vi "Lift.vi"() -> ()   [LabVIEW 2018]
uses:
  <vilib>/Rock Robotics/SystemInterfaces/DIO/FPGA_DIOChannel.ctl
  <vilib>/Rock Robotics/WPI/ThirdParty/Phoenix-LabVIEW/Motor Controller/Controls/CTRE_Phoenix_MotorControl_ControlMode.ctl
  <vilib>/Rock Robotics/WPI/Counter/WPI_CounterDigitalInputToDigitalSource.vi
  Lift Global.vi
  Times/Times Global.vi
  Cargo Intake/Cargo Intake Global.vi
  <vilib>/addons/control/pid/pid.llb/PID (DBL).vi
  <vilib>/addons/control/pid/NI_PID_pid.lvlib
panel:
  in  "LiftMode":T1(ring)
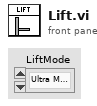
[diagram p1: front panel]
types:
  T1 = enum16{"Ultra Manual Control", "Manual Control", "Basic Control", "Automated Control", "Autonomous Control"}
  T2 = typedef "FPGA_DIOChannel.ctl" = enum8{"DIO 0", "DIO 1", "DIO 2", "DIO 3", "DIO 4", "DIO 5", "DIO 6", "DIO 7", "DIO 8", "DIO 9", "DIO MXP 0", "DIO MXP 1", "DIO MXP 2", "DIO MXP 3", "DIO MXP 4", "DIO MXP 5", "DIO MXP 6", "DIO MXP 7", "DIO MXP 8", "DIO MXP 9", "DIO MXP 10", "DIO MXP 11", "DIO MXP 12", "DIO MXP 13", "DIO MXP 14", "DIO MXP 15", "SPI Port CS1", "SPI Port CS2", "SPI Port CS3", "SPI Port MISO", "SPI Port MOSI", "Invalid"}
  T3 = typedef "WPI_DigitalInputDevRef.ctl" = cluster{"DevStatus":errorcluster, "DIO Channel":T2}
  T4 = enum16{"N/A", "Hatch Panel Zone 1", "Hatch Panel Zone 2", "Hatch Panel Zone 3", "Cargo Zone 1", "Cargo Zone 2", "Cargo Zone 3"}
  T5 = typedef "WPI_MotorControlDeviceRef.ctl" = cluster{"DeviceStatus":errorcluster, "Type":T6, "PWM":cluster{"PWM Channel":T7, "DeadBand":T8}, "CAN":cluster{"Device Number":u8, "SetOutput VI Ref":variant, "GetOutput VI Ref":variant, "Enable VI Ref":variant, "Disable VI Ref":variant, "Data":variant}, "Invert":bool, "DIO PWM":cluster{"PWM \"Enable\" Channel":T7, "DIOChannel":T2, "PWM Rate":dbl}}
  T6 = typedef "WPI_MotorControlType.ctl" = enum16{"PWM", "CAN", "DIO PWM"}
  T7 = typedef "FPGA_DIOPWMChannel.ctl" = enum8{"PWM 0", "PWM 1", "PWM 2", "PWM 3", "PWM 4", "PWM 5", "PWM 6", "PWM 7", "PWM 8", "PWM 9", "PWM MXP 0", "PWM MXP 1", "PWM MXP 2", "PWM MXP 3", "PWM MXP 4", "PWM MXP 5", "PWM MXP 6", "PWM MXP 7", "PWM MXP 8", "PWM MXP 9", "Invalid"}
  T8 = typedef "WPI_PWMDeadband.ctl" = cluster{"Name":string, "maxPositivePwm":i32, "minPositivePwm":i32, "centerPwm":i32, "maxNegativePwm":i32, "minNegativePwm":i32, "angularRange":u16}
  T9 = typedef "CTRE_Phoenix_MotorControl_ControlMode.ctl" = u16
  T10 = typedef "Control 3.ctl" = dbl
  T11 = cluster{"proportional gain (Kc)":dbl, "integral time(Ti, min)":dbl, "derivative time(Td, min) 2":dbl}
  T12 = typedef "FPGA_CounterEncoderSourceConvertionLVSourceType.ctl" = cluster{"DevStatus":errorcluster, "AnalogTriggerMode?":bool, "DigitalMode":cluster{"DIO Channel":T13}, "AnalogTriggerMode":cluster{"AnalogTriggerIndex":T14, "OutputType":T15}}
  T13 = typedef "FPGA_DIODigitalSourceChannel.ctl" = enum8{"DIO 0", "DIO 1", "DIO 2", "DIO 3", "DIO 4", "DIO 5", "DIO 6", "DIO 7", "DIO 8", "DIO 9", "DIO MXP 0", "DIO MXP 1", "DIO MXP 2", "DIO MXP 3", "DIO MXP 4", "DIO MXP 5", "DIO MXP 6", "DIO MXP 7", "DIO MXP 8", "DIO MXP 9", "DIO MXP 10", "DIO MXP 11", "DIO MXP 12", "DIO MXP 13", "DIO MXP 14", "DIO MXP 15", "SPI Port CS1", "SPI Port CS2", "SPI Port CS3", "SPI Port MISO", "SPI Port MOSI", "Disabled"}
  T14 = typedef "FPGA_AnalogTriggerIndex.ctl" = enum8{"Trig 0", "Trig 1", "Trig 2", "Trig 3", "Trig 4", "Trig 5", "Trig 6", "Trig 7", "Invalid"}
  T15 = typedef "FPGA_AnalogTriggerOutType.ctl" = enum16{"InWindow", "TriggerState", "Rising", "Falling"}
  T16 = typedef "WPI_EncoderDevRef.ctl" = cluster{"DevStatus":errorcluster, "EncoderIndex":T17, "CounterIndex":T18, "DistancePerCount":dbl, "Decoding Type":T19}
  T17 = typedef "FPGA_EncoderIdx.ctl" = enum8{"Enc 0", "Enc 1", "Enc 2", "Enc 3", "Enc 4", "Enc 5", "Enc 6", "Enc 7", "Invalid"}
  T18 = typedef "FPGA_CounterCtrSystemIndex.ctl" = enum8{"Ctr 0", "Ctr 1", "Ctr 2", "Ctr 3", "Ctr 4", "Ctr 5", "Ctr 6", "Ctr 7", "Invalid"}
  T19 = typedef "WPI_EncoderType.ctl" = enum16{"1x", "2x", "4x"}
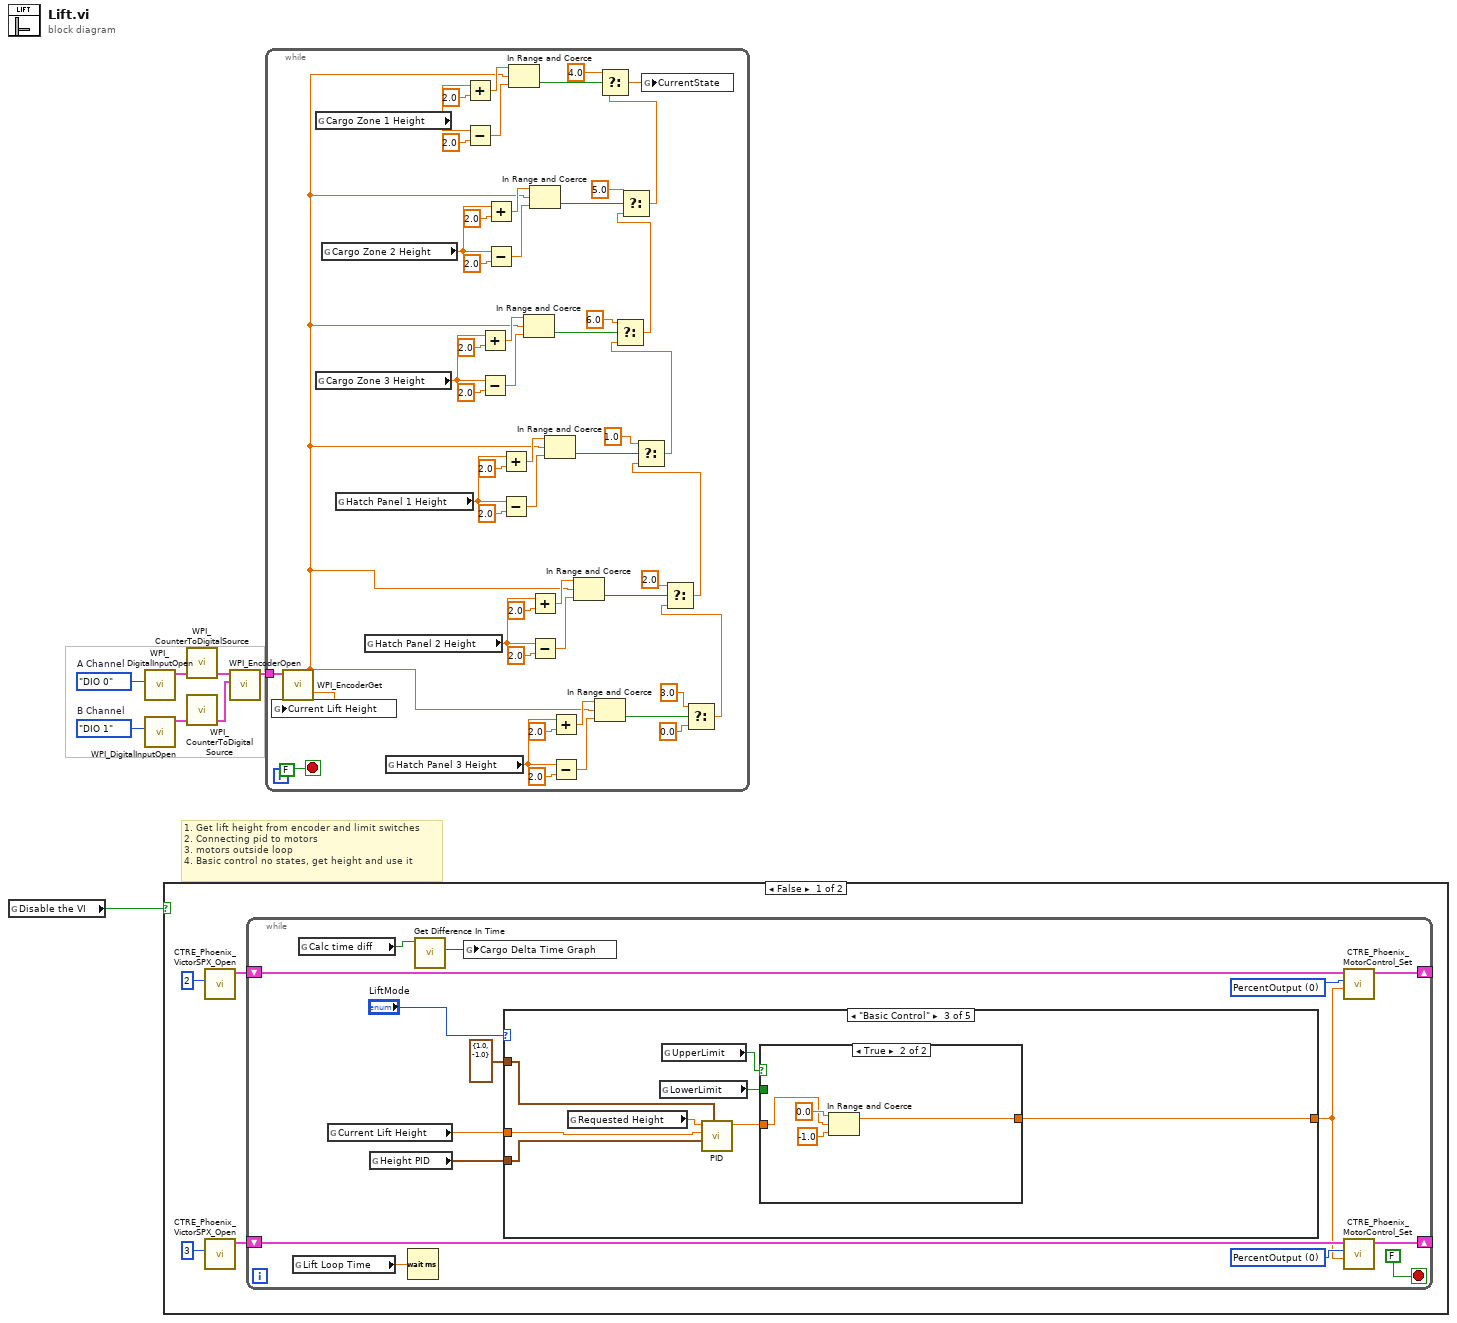
[diagram p0: block diagram]
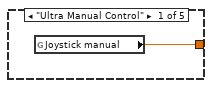
[diagram p2: hidden frame]
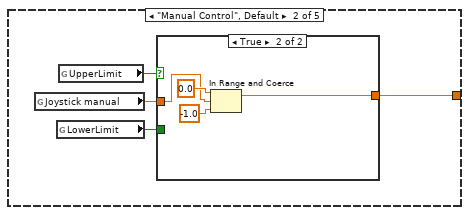
[diagram p3: hidden frame]
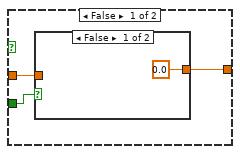
[diagram p4: hidden frame]
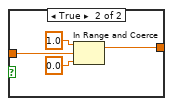
[diagram p5: hidden frame]
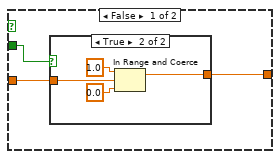
[diagram p6: hidden frame]
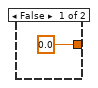
[diagram p7: hidden frame]
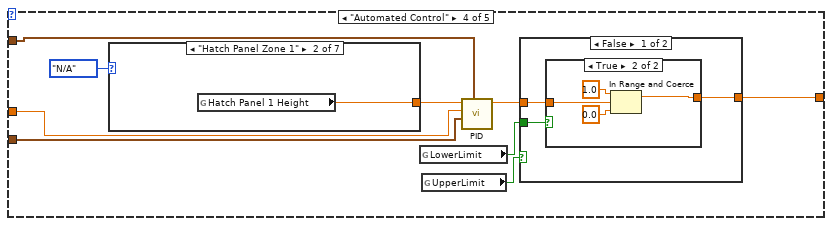
[diagram p8: hidden frame]
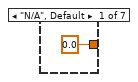
[diagram p9: hidden frame]
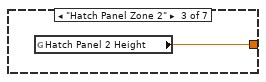
[diagram p10: hidden frame]
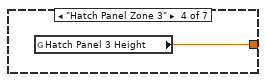
[diagram p11: hidden frame]
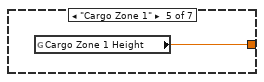
[diagram p12: hidden frame]
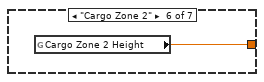
[diagram p13: hidden frame]
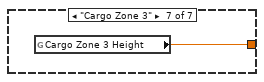
[diagram p14: hidden frame]
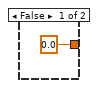
[diagram p15: hidden frame]
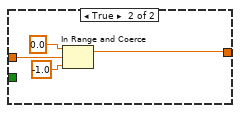
[diagram p16: hidden frame]
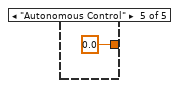
[diagram p17: hidden frame]
diagram:
  w8 = FPGA_DIOChannel."DIO 1"  # B Channel
  w7 = FPGA_DIOChannel."DIO 0"  # A Channel
  # "1. Get lift height from encoder and limit switches\n2. Connecting pid to motors\n3. motors outside loop\n4. Basic control no states, get height and use it"
  n1 = global read "Lift Global.vi" "Disable the VI"() -> (w1:bool)
  n2 = call <vilib>:"WPI_DigitalInputOpen.vi"("DIO Channel"=w7) -> ("DigitalInputDevRef"=w4:T3)  [unwired: 1 in, 9 out]
  n3 = call <vilib>:"WPI_DigitalInputOpen.vi"("DIO Channel"=w8) -> ("DigitalInputDevRef"=w5:T3)  [unwired: 1 in, 9 out]
  n4 = case shown="False" w1 {
    frame False {
      n5 = call <vilib>:"CTRE_Phoenix_VictorSPX_Open.vi"("Device Number"=u8 2) -> ("CAN Talon SRX Ref"=w12:T5)  [unwired: 9 in, 1 out]
      n6 = call <vilib>:"CTRE_Phoenix_VictorSPX_Open.vi"("Device Number"=u8 3) -> ("CAN Talon SRX Ref"=w10:T5)  [unwired: 9 in, 1 out]
      n7 = while {
        shift-right: [w21] -> _
        shift-left: w12 -> [w18]
        shift-right: [w19] -> _
        shift-left: w10 -> [w17]
        stop <- FALSE stop-if-true
        w20 = T9 0 items=["PercentOutput"=0, "Position"=1, "Velocity"=2, "Current"=3, "Follower"=5, "MotionProfile"=6, "MotionMagic"=7, "MotionProfileArc"=10, "Disabled"=15] ("Control Mode")
        w22 = T9 0 items=["PercentOutput"=0, "Position"=1, "Velocity"=2, "Current"=3, "Follower"=5, "MotionProfile"=6, "MotionMagic"=7, "MotionProfileArc"=10, "Disabled"=15] ("Control Mode")
        n8 = global read "Times Global.vi" "Lift Loop Time"() -> (w27:T10)
        n9 = global read "Cargo Intake Global.vi" "Calc time diff"() -> (w24:bool)
        n10 = global read "Lift Global.vi" "Current Lift Height"() -> (w13:dbl)
        n11 = global read "Lift Global.vi" "Height PID"() -> (w14:T11)
        n12 = Wait (ms)(milliseconds to wait=w27) -> ()  [unwired: 1 out]
        n13 = call "Get Difference In Time.vi"("Calculate Time Difference"=w24) -> ("Delta Time over Time"=w23:u32)  [unwired: 9 in, 1 out]
        n14 = global write "Times Global.vi" "Cargo Delta Time Graph"(w23) -> ()
        n15 = case shown="\"Basic Control\"" "LiftMode" {
          tunnel: [w28 w29 w46 w70 0.0 ("Cargo Zone 3 Height")] -> w16
          tunnel: w13 -> [_ _ w52 w68 _]
          tunnel: w14 -> [_ _ w51 w67 _]
          tunnel: cluster{"output high":dbl, "output low":dbl} {"output high"=1.0, "output low"=-1.0} ("output range") -> [_ _ w50 w69 _]
          frame "Ultra Manual Control" {
            n16 = global read "Lift Global.vi" "Joystick manual"() -> (w28:dbl)
          }
          frame "Manual Control", Default {
            n17 = global read "Lift Global.vi" "Joystick manual"() -> (w30:dbl)
            n18 = global read "Lift Global.vi" "LowerLimit"() -> (w32:bool)
            n19 = global read "Lift Global.vi" "UpperLimit"() -> (w31:bool)
            n20 = case shown="True" w31 {
              tunnel: w32 -> [w35 _]
              tunnel: [w34 w42] -> w29
              tunnel: w30 -> [w33 w41]
              frame False {
                n21 = case shown="False" w35 {
                  tunnel: [0.0 w40] -> w34
                  tunnel: w33 -> [_ w37]
                  frame False {
                  }
                  frame True {
                    n22 = In Range and Coerce(upper limit=1.0, x=w37, lower limit=0.0) -> (coerced(x)=w40:dbl)  [unwired: 1 out]
                  }
                }
              }
              frame True {
                n23 = In Range and Coerce(upper limit=0.0, x=w41, lower limit=-1.0) -> (coerced(x)=w42:dbl)  [unwired: 1 out]
              }
            }
          }
          frame "Basic Control" {
            n24 = global read "Lift Global.vi" "Requested Height"() -> (w45:dbl)
            n25 = global read "Lift Global.vi" "LowerLimit"() -> (w49:bool)
            n26 = global read "Lift Global.vi" "UpperLimit"() -> (w48:bool)
            n27 = call-poly <vilib>:"PID.vi"("output range"=w50, "PID gains"=w51, "process variable"=w52, "setpoint"=w45) -> ("output"=w47:dbl)  [unwired: 6 in, 1 out]
            n28 = case shown="True" w48 {
              tunnel: w49 -> [w55 _]
              tunnel: [w54 w62] -> w46
              tunnel: w47 -> [w53 w61]
              frame False {
                n29 = case shown="True" w55 {
                  tunnel: [0.0 w60] -> w54
                  tunnel: w53 -> [_ w57]
                  frame False {
                  }
                  frame True {
                    n30 = In Range and Coerce(upper limit=1.0, x=w57, lower limit=0.0) -> (coerced(x)=w60:dbl)  [unwired: 1 out]
                  }
                }
              }
              frame True {
                n31 = In Range and Coerce(upper limit=0.0, x=w61, lower limit=-1.0) -> (coerced(x)=w62:dbl)  [unwired: 1 out]
              }
            }
          }
          frame "Automated Control" {
            n32 = case shown="\"Hatch Panel Zone 1\"" T4."N/A" ("LiftLocation") {
              tunnel: [0.0 ("Cargo Zone 3 Height") w75 w76 w77 w78 w79 w80] -> w65
              frame "N/A", Default {
              }
              frame "Hatch Panel Zone 1" {
                n33 = global read "Lift Global.vi" "Hatch Panel 1 Height"() -> (w75:dbl)
              }
              frame "Hatch Panel Zone 2" {
                n34 = global read "Lift Global.vi" "Hatch Panel 2 Height"() -> (w76:dbl)
              }
              frame "Hatch Panel Zone 3" {
                n35 = global read "Lift Global.vi" "Hatch Panel 3 Height"() -> (w77:dbl)
              }
              frame "Cargo Zone 1" {
                n36 = global read "Lift Global.vi" "Cargo Zone 1 Height"() -> (w78:dbl)
              }
              frame "Cargo Zone 2" {
                n37 = global read "Lift Global.vi" "Cargo Zone 2 Height"() -> (w79:dbl)
              }
              frame "Cargo Zone 3" {
                n38 = global read "Lift Global.vi" "Cargo Zone 3 Height"() -> (w80:dbl)
              }
            }
            n39 = global read "Lift Global.vi" "LowerLimit"() -> (w73:bool)
            n40 = global read "Lift Global.vi" "UpperLimit"() -> (w72:bool)
            n41 = call-poly <vilib>:"PID.vi"("output range"=w69, "PID gains"=w67, "process variable"=w68, "setpoint"=w65) -> ("output"=w71:dbl)  [unwired: 6 in, 1 out]
            n42 = case shown="False" w72 {
              tunnel: w73 -> [w83 _]
              tunnel: [w82 w90] -> w70
              tunnel: w71 -> [w81 w89]
              frame False {
                n43 = case shown="True" w83 {
                  tunnel: [0.0 w88] -> w82
                  tunnel: w81 -> [_ w85]
                  frame False {
                  }
                  frame True {
                    n44 = In Range and Coerce(upper limit=1.0, x=w85, lower limit=0.0) -> (coerced(x)=w88:dbl)  [unwired: 1 out]
                  }
                }
              }
              frame True {
                n45 = In Range and Coerce(upper limit=0.0, x=w89, lower limit=-1.0) -> (coerced(x)=w90:dbl)  [unwired: 1 out]
              }
            }
          }
          frame "Autonomous Control" {
          }
        }
        n46 = call <vilib>:"CTRE_Phoenix_MotorControl_Set.vi"("Output"=w16, "Control Mode"=w22, "PhoenixMotorControlDevRef"=w18) -> ("PhoenixMotorControlDevRef"=w21:T5)  [unwired: 7 in, 1 out]
        n47 = call <vilib>:"CTRE_Phoenix_MotorControl_Set.vi"("Output"=w16, "Control Mode"=w20, "PhoenixMotorControlDevRef"=w17) -> ("PhoenixMotorControlDevRef"=w19:T5)  [unwired: 7 in, 1 out]
      }
    }
    frame True {
    }
  }
  n48 = call-poly <vilib>:"WPI_CounterToDigitalSource.vi"("DigitalInputDevRef"=w4) -> ("Digital Source"=w3:T12)  [unwired: 6 out]
  n49 = call-poly <vilib>:"WPI_CounterToDigitalSource.vi"("DigitalInputDevRef"=w5) -> ("Digital Source"=w6:T12)  [unwired: 6 out]
  n50 = call <vilib>:"WPI_EncoderOpen.vi"("BSource"=w6, "ASource"=w3) -> ("EncoderDevRef"=w2:T16)  [unwired: 6 in, 3 out]
  n51 = while {
    tunnel: w2 -> [w145]
    stop <- FALSE stop-if-true
    n52 = call <vilib>:"WPI_EncoderGet.vi"("EncoderDevRef"=w145) -> ("Distance"=w94:dbl)  [unwired: 5 in, 5 out]
    n53 = global write "Lift Global.vi" "Current Lift Height"(w94) -> ()
    n54 = global read "Lift Global.vi" "Cargo Zone 1 Height"() -> (w134:dbl)
    n55 = global read "Lift Global.vi" "Cargo Zone 3 Height"() -> (w122:dbl)
    n56 = global read "Lift Global.vi" "Cargo Zone 2 Height"() -> (w140:dbl)
    n57 = global read "Lift Global.vi" "Hatch Panel 1 Height"() -> (w128:dbl)
    n58 = global read "Lift Global.vi" "Hatch Panel 2 Height"() -> (w110:dbl)
    n59 = global read "Lift Global.vi" "Hatch Panel 3 Height"() -> (w116:dbl)
    n60 = Add(x=w134, y=2.0) -> (x+y=w136:dbl)
    n61 = Subtract(x=w134, y=2.0) -> (x-y=w137:dbl)
    n62 = Add(x=w122, y=2.0) -> (x+y=w124:dbl)
    n63 = Subtract(x=w122, y=2.0) -> (x-y=w125:dbl)
    n64 = Add(x=w140, y=2.0) -> (x+y=w142:dbl)
    n65 = Subtract(x=w140, y=2.0) -> (x-y=w143:dbl)
    n66 = Add(x=w128, y=2.0) -> (x+y=w130:dbl)
    n67 = Subtract(x=w128, y=2.0) -> (x-y=w131:dbl)
    n68 = In Range and Coerce(upper limit=w136, x=w94, lower limit=w137) -> (In Range?=w132:bool)  [unwired: 1 out]
    n69 = In Range and Coerce(upper limit=w124, x=w94, lower limit=w125) -> (In Range?=w120:bool)  [unwired: 1 out]
    n70 = In Range and Coerce(upper limit=w142, x=w94, lower limit=w143) -> (In Range?=w138:bool)  [unwired: 1 out]
    n71 = Add(x=w110, y=2.0) -> (x+y=w112:dbl)
    n72 = Subtract(x=w110, y=2.0) -> (x-y=w113:dbl)
    n73 = In Range and Coerce(upper limit=w130, x=w94, lower limit=w131) -> (In Range?=w126:bool)  [unwired: 1 out]
    n74 = Add(x=w116, y=2.0) -> (x+y=w118:dbl)
    n75 = Subtract(x=w116, y=2.0) -> (x-y=w119:dbl)
    n76 = In Range and Coerce(upper limit=w112, x=w94, lower limit=w113) -> (In Range?=w108:bool)  [unwired: 1 out]
    n77 = In Range and Coerce(upper limit=w118, x=w94, lower limit=w119) -> (In Range?=w114:bool)  [unwired: 1 out]
    n78 = Select(t=3.0, s=w114, f=0.0 ("t")) -> (s? t:f=w104:dbl)
    n79 = Select(t=2.0, s=w108, f=w104) -> (s? t:f=w105:dbl)
    n80 = Select(t=1.0, s=w126, f=w105) -> (s? t:f=w106:dbl)
    n81 = Select(t=6.0, s=w120, f=w106) -> (s? t:f=w107:dbl)
    n82 = Select(t=5.0, s=w138, f=w107) -> (s? t:f=w101:dbl)
    n83 = Select(t=4.0, s=w132, f=w101) -> (s? t:f=w102:dbl)
    n84 = global write "Lift Global.vi" "CurrentState"(w102) -> ()
  }
